vi "RomiSim_Create_Model.vi"(11 "Initial Robot Position":T1={"TRANSLATION"={"X"=0.0, "Y"=0.0}, "ROTATION"={"VALUE"=0.0, "COS"=1.0, "SIN"=0.0}} {"ROTATION"."SIN" format="%13.4f"; "ROTATION"."COS" format="%13.4f"; "ROTATION"."VALUE" format="%13.4f"; "TRANSLATION"."Y" format="%14.3f"; "TRANSLATION"."X" format="%14.3f"}) -> (2 "Encoder Ft/Count":dbl, 3 "out DiffDriveTrainSim":T4 {"m_Motor"."Jr_KgM2" format="%13.5p"; "m_Motor"."L_H" format="%13.5p"; "m_Motor"."Kt_NMPerAmp" format="%13.5p"; "m_Motor"."KvINV_RadPerSecPerVolt" format="%13.5p"; "m_Motor"."R_Ohms" format="%13.5p"; "m_Motor"."FreeSpeed_RadPerSec" format="%13.5p"; "m_Motor"."FreeCurrent_Amps" format="%13.5p"; "m_Motor"."StallCurrent_Amps" format="%13.5p"; "m_Motor"."StallTorque_NM" format="%13.5p"; "m_Motor"."nominalVoltage_Volts" format="%13.5p"})   [LabVIEW 2019]
uses:
  <vilib>/Rock Robotics/WPI/ThirdParty/JAS_Junk/TrajLib/Trajectory_Library.lvlib
  <vilib>/Rock Robotics/WPI/ThirdParty/JAS_Junk/TrajLib/Enum/DCMOTOR_TYPES_ENUM.ctl
  <vilib>/Analysis/Matrix/Datatypes/RealMatrix.ctl
  <vilib>/Analysis/Matrix/NI_Matrix.lvlib
  <vilib>/Rock Robotics/WPI/ThirdParty/JAS_Junk/TrajLib/TypeDef/LINEAR_SYSTEM.ctl
  <vilib>/Rock Robotics/WPI/ThirdParty/JAS_Junk/TrajLib/TypeDef/DCMOTOR.CTL
  <vilib>/Rock Robotics/WPI/ThirdParty/JAS_Junk/TrajLib/TypeDef/DIFF_DRIVE_TRAIN_SIM.ctl
  <vilib>/Rock Robotics/WPI/ThirdParty/JAS_Junk/TrajLib/TypeDef/TRANSLATION2D.ctl
  <vilib>/Rock Robotics/WPI/ThirdParty/JAS_Junk/TrajLib/TypeDef/ROTATION2D.ctl
  <vilib>/Rock Robotics/WPI/ThirdParty/JAS_Junk/TrajLib/TypeDef/POSE2D.ctl
panel:
  # "<States, 1>"
  # "<Outputs, 1>"
  # "<Inputs, 1>"
  # "<Outputs, 1>"
  # "<States,States>"
  # "<States,Inputs>"
  # "<Outputs,States>"
  # "<Outputs,Inputs>"
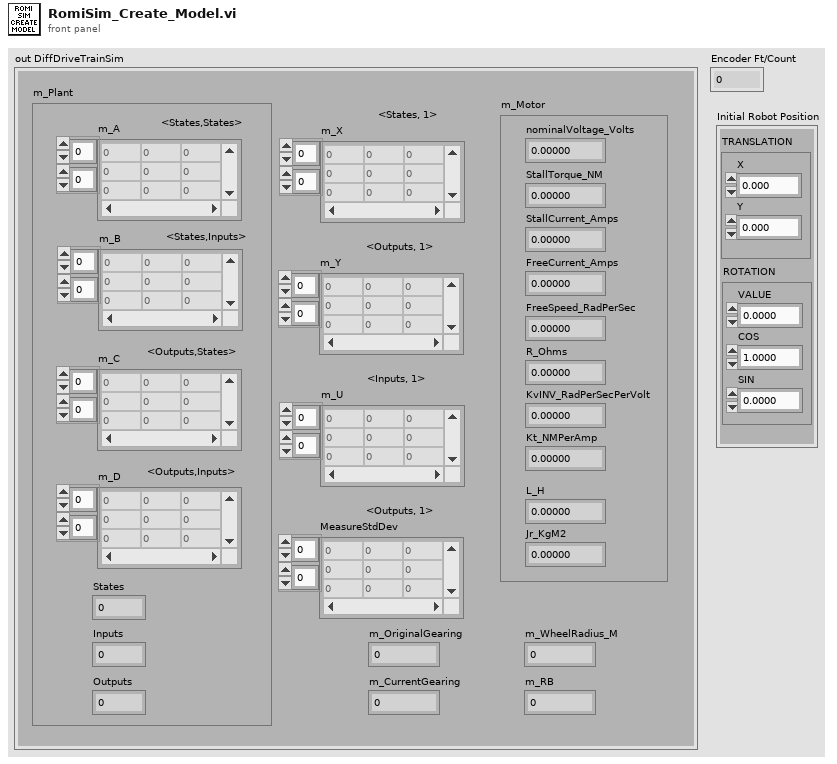
[diagram p1: front panel]
types:
  T1 = typedef "Trajectory_Library.lvlib/POSE2D.ctl" = cluster{"TRANSLATION":T2, "ROTATION":T3}
  T2 = typedef "Trajectory_Library.lvlib/TRANSLATION2D.ctl" = cluster{"X":dbl, "Y":dbl}
  T3 = typedef "Trajectory_Library.lvlib/ROTATION2D.ctl" = cluster{"VALUE":dbl, "COS":dbl, "SIN":dbl}
  T4 = typedef "Trajectory_Library.lvlib/DIFF_DRIVE_TRAIN_SIM.ctl" = cluster{"m_Plant":T5, "m_X":T6, "m_Y":T6, "m_U":T6, "MeasureStdDev":T6, "m_Motor":T7, "m_OriginalGearing":dbl, "m_CurrentGearing":dbl, "m_WheelRadius_M":dbl, "m_RB":dbl}
  T5 = typedef "Trajectory_Library.lvlib/LINEAR_SYSTEM.ctl" = cluster{"m_A":T6, "m_B":T6, "m_C":T6, "m_D":T6, "States":i32, "Inputs":i32, "Outputs":i32}
  T6 = typedef "NI_Matrix.lvlib/RealMatrix.ctl" = dbl[][]
  T7 = typedef "Trajectory_Library.lvlib/DCMOTOR.CTL" = cluster{"nominalVoltage_Volts":dbl, "StallTorque_NM":dbl, "StallCurrent_Amps":dbl, "FreeCurrent_Amps":dbl, "FreeSpeed_RadPerSec":dbl, "R_Ohms":dbl, "KvINV_RadPerSecPerVolt":dbl, "Kt_NMPerAmp":dbl, "L_H":dbl, "Jr_KgM2":dbl}
  T8 = typedef "Trajectory_Library.lvlib/DCMOTOR_TYPES_ENUM.ctl" = enum16{"CIM", "AndyMark 9015", "Andy Mark RS 775 125", "Bag", "BaneBots RS 550", "BaneBots RS 775", "Falcon 500", "Mini CIM", "NEO", "NEO 550", "Romi BuiltIn", "Vex 775 Pro"}
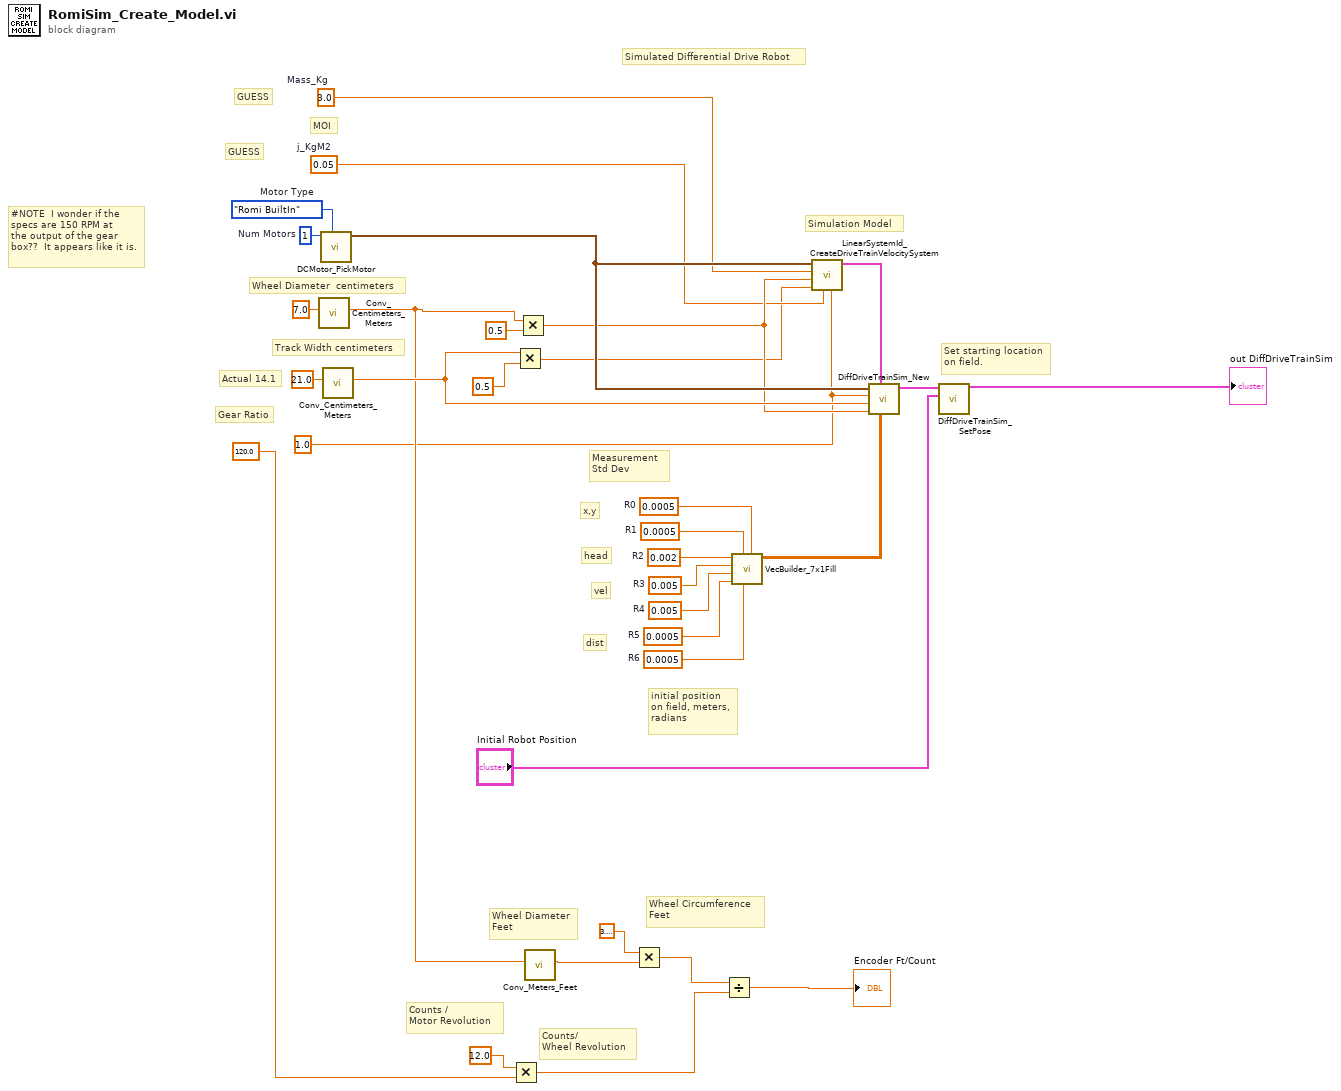
[diagram p0: block diagram]
diagram:
  w2 = 1.0 ("INCH")
  w27 = 1  # Num Motors
  w28 = DCMOTOR_TYPES_ENUM."Romi BuiltIn"  # Motor Type
  w21 = 3.0  # Mass_Kg
  w23 = 0.05  # j_KgM2
  w12 = 0.0005  # R6
  w13 = 0.0005  # R5
  w14 = 0.005  # R4
  w15 = 0.005  # R3
  w16 = 0.002  # R2
  w17 = 0.0005  # R1
  w18 = 0.0005  # R0
  # "Actual 14.1"
  # "#NOTE  I wonder if the \nspecs are 150 RPM at\nthe output of the gear\nbox??  It appears like it is."
  # "Wheel Circumference\nFeet"
  # "Wheel Diameter\nFeet"
  # "Counts/\nWheel Revolution"
  # "Counts /\nMotor Revolution"
  # "Set starting location\non field."
  # "Measurement \nStd Dev"
  # "Gear Ratio"
  # "GUESS"
  # "GUESS"
  # "Track Width centimeters"
  # "Wheel Diameter  centimeters"
  # "MOI"
  # "dist"
  # "vel"
  # "head"
  # "x,y"
  # "Simulated Differential Drive Robot"
  # "initial position\non field, meters,\nradians"
  # "Simulation Model"
  n1 = call <vilib>:"Conv_Centimeters_Meters.vi"("Centimeter"=7.0 ("INCH")) -> ("Meters"=w9:dbl)  [unwired: 10 in]
  n2 = call <vilib>:"DCMotor_PickMotor.vi"("DCMOTOR_TYPES"=w28, "Num Motors"=w27) -> ("DCMOTOR"=w29:T7)  [unwired: 9 in]
  n3 = call <vilib>:"Conv_Centimeters_Meters.vi"("Centimeter"=21.0 ("INCH")) -> ("Meters"=w30:dbl)  [unwired: 10 in]
  n4 = Multiply(x=12.0, y=120.0 ("INCH")) -> (x*y=w8:dbl)
  n5 = Multiply(x=w30, y=0.5) -> (x*y=w22:dbl)
  n6 = Multiply(x=w9, y=0.5) -> (x*y=w24:dbl)
  n7 = call <vilib>:"Conv_Meters_Feet.vi"("Meters"=w9) -> ("Feet"=w6:dbl)  [unwired: 10 in]
  n8 = Multiply(x=3.141592653589793, y=w6) -> (x*y=w5:dbl)
  n9 = Divide(x=w5, y=w8) -> (x/y=→"Encoder Ft/Count":dbl)
  n10 = call <vilib>:"VecBuilder_7x1Fill.vi"("R0"=w18, "R6"=w12, "R1"=w17, "R5"=w13, "R4"=w14, "R3"=w15, "R2"=w16) -> ("output matrix"=w32:T6)  [unwired: 4 in]
  n11 = call <vilib>:"LinearSystemId_CreateDriveTrainVelocitySystem.vi"("G"=w2, "JKgMetersSquared"=w23, "rbMeters"=w22, "rMeters"=w24, "MassKg"=w21, "Motor"=w29) -> ("Linearsystem"=w20:T5)  [unwired: 4 in, 1 out]
  n12 = call <vilib>:"DiffDriveTrainSim_New.vi"("MeasurementStdDev"=w32, "DriveTrainPlant"=w20, "WheelRadius_M"=w24, "TrackWidth_M"=w30, "Gearing"=w2, "DriveMotor"=w29) -> ("DiffDriveTrainSim"=w33:T4)  [unwired: 5 in]
  n13 = call <vilib>:"DiffDriveTrainSim_SetPose.vi"("Pose"="Initial Robot Position", "in DiffDriveTrainSim"=w33) -> ("out DiffDriveTrainSim"=→"out DiffDriveTrainSim":T4)  [unwired: 9 in]
